vi "Send.vi"(8 "error in (no error)":errorcluster, 9 "Queue":refnum<class "Message Enqueuer.lvclass">, 10 "Data":cluster{"EDR":dbl, "Pulse":u8}, 11 "Data Update Msg in":refnum<class "Data Update Msg.lvclass">) -> (0 "error out":errorcluster, 3 "Data Update Msg out":refnum<class "Data Update Msg.lvclass">)   [LabVIEW 2011, in "Data Update Msg.lvclass"]
uses:
  Data Update Msg.lvclass
  <userlib>/_Frameworks/ActorFramework/Message Enqueuer/Message Enqueuer.lvclass
  Data Update Msg.lvclass/Data Update Msg.ctl
  <userlib>/_Frameworks/ActorFramework/Message Enqueuer/Message Enqueuer.lvclass/Message Enqueuer.ctl
  <userlib>/_Frameworks/ActorFramework/Message Priority Queue/Priority Enqueue.vi
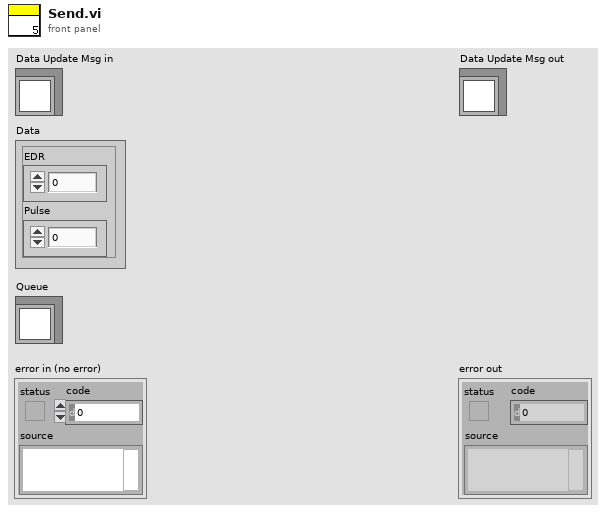
[diagram p1: front panel]
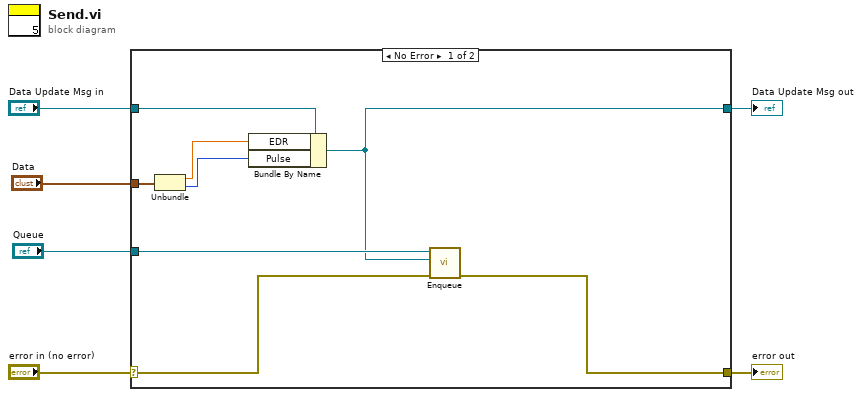
[diagram p0: block diagram]
diagram:
  n1 = case shown="No Error" "error in (no error)" {
    selector: "error in (no error)" -> [w8 w16]
    tunnel: [w7 w16] -> w5
    tunnel: [w9 w15] -> w3
    tunnel: "Data Update Msg in" -> [w14 w15]
    tunnel: "Data" -> [w13 _]
    tunnel: "Queue" -> [w10 _]
    frame No Error {
      n2 = Unbundle(w13) -> ("EDR"=w12:dbl, "Pulse"=w11:u8)
      n3 = Bundle By Name(cluster=w14, "EDR"=w12, "Pulse"=w11) -> (w9:refnum<class "Data Update Msg.lvclass">)
      n4 = call <userlib>:"Enqueue.vi"("error in (no error)"=w8, "Message"=w9, "Message Enqueuer in"=w10) -> ("error out"=w7:errorcluster)  [unwired: 7 in, 1 out]
    }
    frame Error {
    }
  }
  "error out" <- w5
  "Data Update Msg out" <- w3
